vi "Returning A Value Array Of Integers.vi"(11 "length":i32) -> (3 "function return":i32)   [LabVIEW 2018, in "ParsingDataSampleDLL.lvlib"]
doc: "__declspec(dllexport) int* ReturningAValue_ArrayOfIntegers (int length);"
uses:
  ParsingDataSampleDLL.lvlib
  ni_reference_vs/Debug/ParsingDataSampleDLL.dll
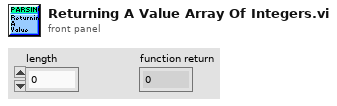
[diagram p1: front panel]
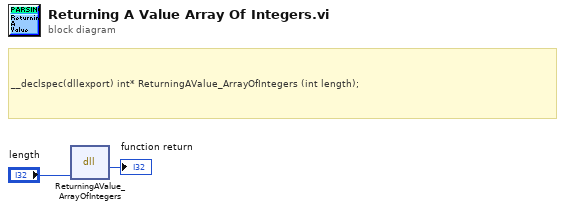
[diagram p0: block diagram]
diagram:
  # "__declspec(dllexport) int* ReturningAValue_ArrayOfIntegers (int length);"
  n1 = dll-call lib="C:/Users/celit/Documents/GitHub/Labview_Python_DLL_Call/ni_reference_vs/Debug/ParsingDataSampleDLL.*" fn="ReturningAValue_ArrayOfIntegers"("length"="length") -> (→"function return":i32)  [unwired: 4 in, 2 out]
